vi "Sensor_Values.vi"() -> ()   [LabVIEW 2019]
panel:
  in  "Drive_IMU (deg)":dbl
  in  "Back_Right_Wheel_Angle (deg)":dbl
  in  "Back_Left_Wheel_Angle (deg)":dbl
  in  "Front_Left_Wheel_Angle (deg)":dbl
  in  "Front_Right_Wheel_Angle (deg)":dbl
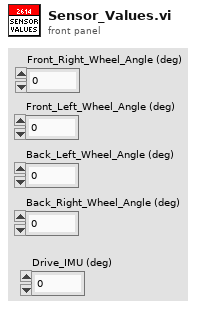
[diagram p1: front panel]
diagram:
